vi "Step Add GND W Parameters.vi"(0 "VISA resource name":refnum<visa-resource-name>, 1 "Scanner Channel (0 - 16) (0)":u32, 2 "Internal Scanner Exists?":bool, 5 "GND Test Paramameters":T1={"Current (1 - 32 A) (25A)"=25.0, "Voltage (3 - 8 V) (8V)"=8.0, "High Limit (0 - 200 mohm)(100 mohm)"=100, "Low Limit (0 - 200 mohm)(0 mohm)"=0, "High Limit V (0 - 6.00 V) (6V)"=6.0, "Low Limit V (0 - 6.00 V) (0V)"=0.0, "Dwell Time (0.0, 0.5 - 999.9 s) (1.0S)"=1.0, "Offset (0 - 200 mohm) (0mohm)"=0, "Offset V (0 - 6.00 V) (0V)"=0.0, "Frequency (50/60 HZ) (50HZ)"=enum."50", "Auto Offset (F: Off)"=FALSE} {"Offset V (0 - 6.00 V) (0V)" format="%#.2f"; "Dwell Time (0.0, 0.5 - 999.9 s) (1.0S)" format="%.1f"; "Low Limit V (0 - 6.00 V) (0V)" format="%#.2f"; "High Limit V (0 - 6.00 V) (6V)" format="%#.2f"; "Voltage (3 - 8 V) (8V)" format="%.2f"; "Current (1 - 32 A) (25A)" format="%.2f"}, 7 "Step Selection (1-200)":i32=1, 9 "Add Step":bool, 11 "error in (no error)":errorcluster) -> (4 "VISA resource name out":refnum<visa-resource-name>, 15 "error out":errorcluster)   [LabVIEW 2020, in "Associated Research 78XX Series.lvlib"]
doc: "Sets the parameters for the CONT test mode for the given memory location."
uses:
  <instrlib>/Associated Research 78XX Series/Associated Research 78XX Series.lvlib
  <instrlib>/Associated Research 78XX Series/Public/Configure/Steps/Low Level/GND Test Parameters.ctl
panel:
  # "NOTE:\nFirmware version greater than 2.00.00, the following parameters are workable.\nHigh Limit V (0 - 6.00 V)\nLow Limit V (0 - 6.00 V)\nOffset V (0 - 6.00 V)"
  # "Add"
  # "Edit"
  # "On\nOff"
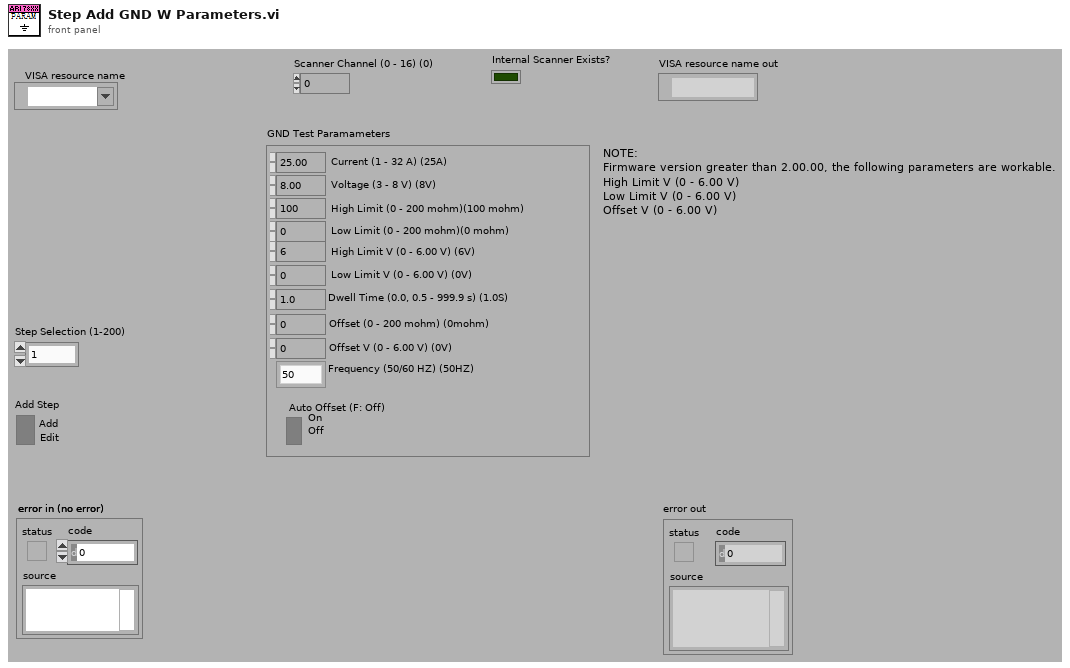
[diagram p1: front panel]
types:
  T1 = typedef "Associated Research 78XX Series.lvlib/GND Test Parameters.ctl" = cluster{"Current (1 - 32 A) (25A)":dbl, "Voltage (3 - 8 V) (8V)":dbl, "High Limit (0 - 200 mohm)(100 mohm)":i32, "Low Limit (0 - 200 mohm)(0 mohm)":i32, "High Limit V (0 - 6.00 V) (6V)":dbl, "Low Limit V (0 - 6.00 V) (0V)":dbl, "Dwell Time (0.0, 0.5 - 999.9 s) (1.0S)":dbl, "Offset (0 - 200 mohm) (0mohm)":i32, "Offset V (0 - 6.00 V) (0V)":dbl, "Frequency (50/60 HZ) (50HZ)":enum16{"50", "60"}, "Auto Offset (F: Off)":bool}
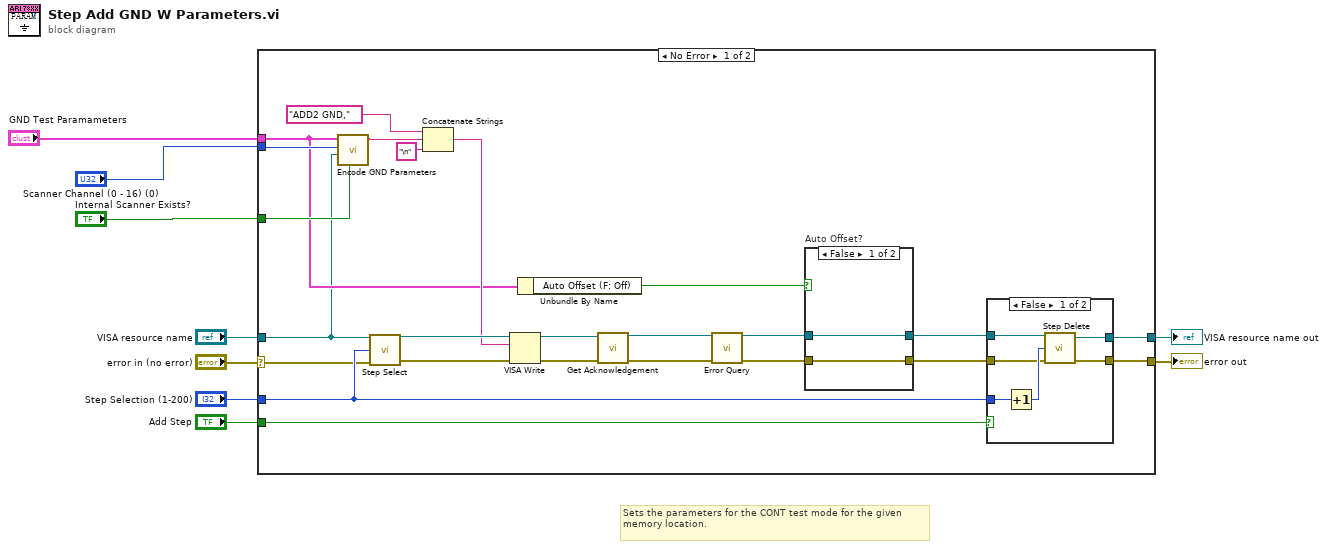
[diagram p0: block diagram]
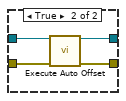
[diagram p2: hidden frame]
diagram:
  # "Sets the parameters for the CONT test mode for the given memory location."
  n1 = case shown="No Error" "error in (no error)" {
    selector: "error in (no error)" -> [w11 w49]
    tunnel: [w31 w49] -> w8
    tunnel: [w30 w48] -> w6
    tunnel: "VISA resource name" -> [w10 w48]
    tunnel: "Step Selection (1-200)" -> [w19 _]
    tunnel: "Add Step" -> [w29 _]
    tunnel: "GND Test Paramameters" -> [w12 _]
    tunnel: "Internal Scanner Exists?" -> [w15 _]
    tunnel: "Scanner Channel (0 - 16) (0)" -> [w14 _]
    frame No Error {
      n2 = call <instrlib>:"Encode GND Parameters.vi"("Internal Scanner Exists?"=w15, "VISA resource name"=w10, "Scanner Channel (0 - 16) (0=Off)"=w14, "GND Test Paramameters"=w12) -> ("Add Step"=w16:string)  [unwired: 5 in, 2 out]
      n3 = call <instrlib>:"Step Select.vi"("VISA resource name"=w10, "Step Number (1)"=w19, "error in (no error)"=w11) -> ("VISA resource name out"=w32:refnum<visa-resource-name>, "error out"=w33:errorcluster)  [unwired: 11 in]
      n4 = Concatenate Strings("ADD2 GND," ("string"), w16, "\n" ("string")) -> (w13:string)
      n5 = VISA Write(VISA resource name=w32, write buffer=w13, error in (no error)=w33) -> (VISA resource name out=w18:refnum<visa-resource-name>, error out=w17:errorcluster)  [unwired: 1 out]
      n6 = Unbundle By Name(w12) -> ("Auto Offset (F: Off)"=w23:bool)
      n7 = call <instrlib>:"Get Acknowledgement.vi"("VISA resource name"=w18, "error in (no error)"=w17) -> ("VISA resource name out"=w22:refnum<visa-resource-name>, "error out"=w21:errorcluster)  [unwired: 12 in]
      n8 = call <instrlib>:"Error Query.vi"("VISA resource name"=w22, "error in (no error)"=w21) -> ("VISA resource name out"=w27:refnum<visa-resource-name>, "error out"=w26:errorcluster)  [unwired: 10 in, 2 out]
      n9 = case "Auto Offset?" shown="False" w23 {
        tunnel: w27 -> [w35 w39]
        tunnel: w26 -> [w34 w38]
        tunnel: [w34 w36] -> w25
        tunnel: [w35 w37] -> w24
        frame False {
        }
        frame True {
          n10 = call <instrlib>:"Execute Auto Offset.vi"("VISA resource name"=w39, "error in (no error)"=w38) -> ("VISA resource name out"=w37:refnum<visa-resource-name>, "error out"=w36:errorcluster)  [unwired: 12 in]
        }
      }
      n11 = case shown="False" w29 {
        tunnel: w19 -> [w45 _]
        tunnel: w25 -> [w43 w46]
        tunnel: w24 -> [w42 w47]
        tunnel: [w41 w46] -> w31
        tunnel: [w40 w47] -> w30
        frame False {
          n12 = Increment(x=w45) -> (x+1=w44:i32)
          n13 = call <instrlib>:"Step Delete.vi"("VISA resource name"=w42, "Step Number (0 = Active Step)"=w44, "error in (no error)"=w43) -> ("VISA resource name out"=w40:refnum<visa-resource-name>, "error out"=w41:errorcluster)  [unwired: 11 in]
        }
        frame True {
        }
      }
    }
    frame Error {
    }
  }
  "error out" <- w8
  "VISA resource name out" <- w6
